vi "TON ONS.vi"(9 "Delay (ms)":u32=500, 10 "Input":bool) -> (2 "Output 2":bool)   [LabVIEW 2014]
panel:
  out "Last State":bool
  in  "Delay_TON":T1
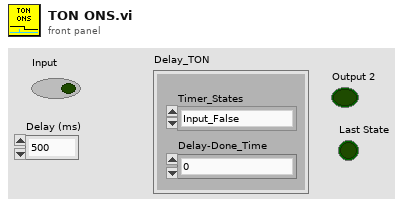
[diagram p1: front panel]
types:
  T1 = cluster{"Timer_States":enum16{"Input_False", "Input_True_Start_Timing", "Input_True_Timing", "Input_True_Timing_Complete"}, "Delay-Done_Time":u32}
  T2 = enum16{"Input_False", "Input_True_Start_Timing", "Input_True_Timing", "Input_True_Timing_Complete"}
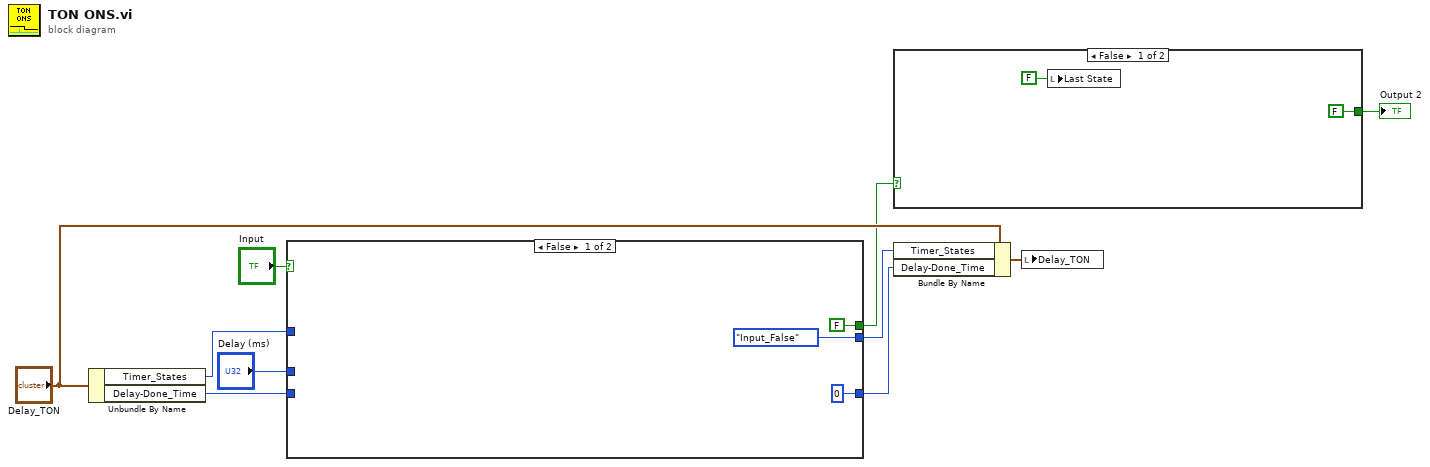
[diagram p0: block diagram]
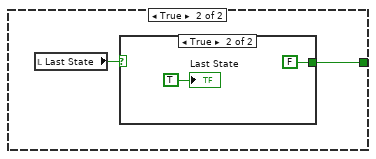
[diagram p2: hidden frame]
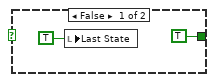
[diagram p3: hidden frame]
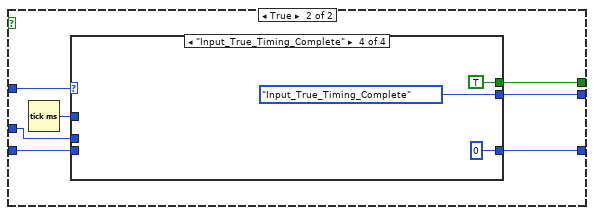
[diagram p4: hidden frame]
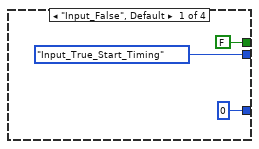
[diagram p5: hidden frame]
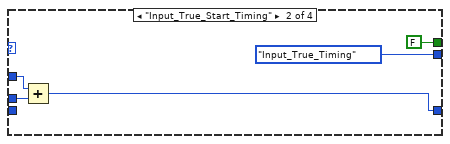
[diagram p6: hidden frame]
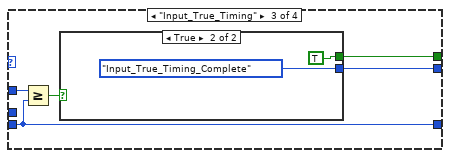
[diagram p7: hidden frame]
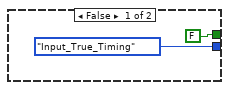
[diagram p8: hidden frame]
diagram:
  n1 = Unbundle By Name("Delay_TON") -> ("Timer_States"=w9:T2, "Delay-Done_Time"=w5:u32)
  n2 = case shown="False" "Input" {
    tunnel: [FALSE ("Boolean 2") w15] -> w1
    tunnel: w9 -> [_ w14]
    tunnel: [T2."Input_False" ("Timer_States") w20] -> w8
    tunnel: [u32 0 ("Delay-Done_Time") w19] -> w7
    tunnel: "Delay (ms)" -> [_ w17]
    tunnel: w5 -> [_ w16]
    frame False {
    }
    frame True {
      n3 = Tick Count (ms)() -> (millisecond timer value=w18:u32)
      n4 = case shown="\"Input_True_Timing_Complete\"" w14 {
        tunnel: [T2."Input_True_Start_Timing" ("Timer_States") T2."Input_True_Timing" ("Timer_States") w31 T2."Input_True_Timing_Complete" ("Timer_States")] -> w20
        tunnel: [u32 0 ("Delay-Done_Time") w26 w29 u32 0 ("Delay-Done_Time")] -> w19
        tunnel: w18 -> [_ w28 w33 _]
        tunnel: w17 -> [_ w27 _ _]
        tunnel: w16 -> [_ _ w29 _]
        tunnel: [FALSE ("DOUT-TON") FALSE ("DOUT-TON") w30 TRUE ("DOUT-TON")] -> w15
        frame "Input_False", Default {
        }
        frame "Input_True_Start_Timing" {
          n5 = Add(x=w28, y=w27) -> (x+y=w26:u32)
        }
        frame "Input_True_Timing" {
          n6 = Greater Or Equal?(x=w33, y=w29) -> (x >= y?=w32:bool)
          n7 = case shown="True" w32 {
            tunnel: [T2."Input_True_Timing" ("Timer_States") T2."Input_True_Timing_Complete" ("Timer_States")] -> w31
            tunnel: [FALSE TRUE] -> w30
            frame False {
            }
            frame True {
            }
          }
        }
        frame "Input_True_Timing_Complete" {
        }
      }
    }
  }
  n8 = case shown="False" w1 {
    tunnel: [FALSE ("One-Shot Output") w44] -> w2
    frame False {
      n9 = local write "Last State"(FALSE ("Last State")) -> ()
    }
    frame True {
      n10 = local read "Last State"() -> (w43:bool)
      n11 = case shown="True" w43 {
        tunnel: [TRUE ("One-Shot Output") FALSE ("One-Shot Output")] -> w44
        frame False {
          n12 = local write "Last State"(TRUE ("Last State")) -> ()
        }
        frame True {
          "Last State" <- TRUE ("Last State")
        }
      }
    }
  }
  "Output 2" <- w2
  n13 = Bundle By Name(cluster="Delay_TON", "Timer_States"=w8, "Delay-Done_Time"=w7) -> (w3:T1)
  n14 = local write "Delay_TON"(w3) -> ()
